vi "mainSystem.vi"() -> ()   [LabVIEW 2012, in "GUILib.lvlib"]
doc: "example for a main (top) system"
uses:
  GUILib.lvlib
  GUILib.userEventsMainType.ctl
  UtilityLib/UtilityLib.valueStatus.ctl
  UtilityLib/UtilityLib.lvlib
panel:
  in  "stop":bool
  in  "userEventsMain":T1
  in  "subSystem3":bool
  in  "userEvent":refnum<user-event>
  in  "subSystem2":bool
  in  "subSystem1":bool
  out "subSystem1state":bool
  out "subSystem3state":bool
  out "subSystem2state":bool
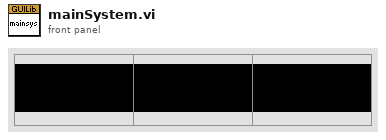
[diagram p1: front panel]
types:
  T1 = typedef "GUILib.lvlib/GUILib.userEventsMainType.ctl" = cluster{"data":string, "dataType":i32}
  T2 = typedef "UtilityLib.lvlib/UtilityLib.valueStatus.ctl" = enum16{"no info available", "stand by/off", "on", "warning", "alarm/malfunction", "not implemented", "user action required", "important information", "system default", "control default", "indicator default", "button default"}
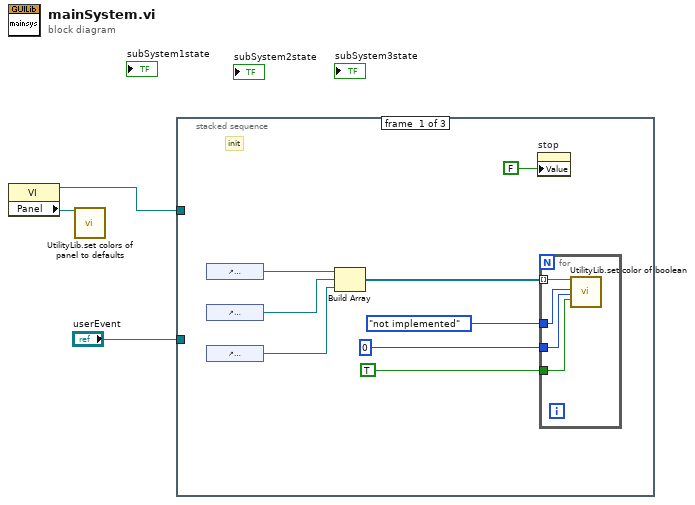
[diagram p0: block diagram]
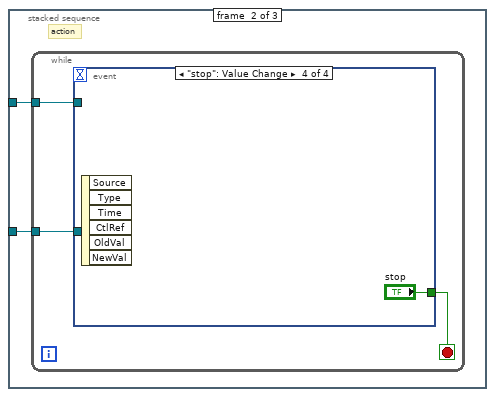
[diagram p2: hidden frame]
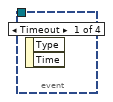
[diagram p3: hidden frame]
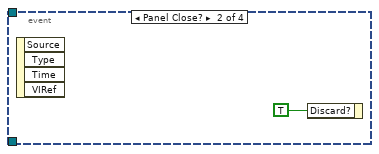
[diagram p4: hidden frame]
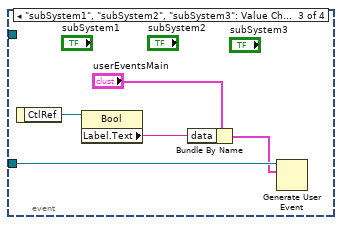
[diagram p5: hidden frame]
diagram:
  n1 = property on="Property Node" class="VI"() -> (reference out=w1:refnum<vi>, "Panel"=w2:refnum<vi>)  [unwired: 2 in, 1 out]
  n2 = call "UtilityLib.set colors of panel to defaults.vi"("Front Panel"=w2) -> ()  [unwired: 18 in, 1 out]
  n3 = stacked-sequence {
    tunnel: "userEvent" -> [_ w17 _]
    tunnel: w1 -> [_ w16 _]
    frame #0 {
      # "init"
      n4 = control-ref of="subSystem1state"() -> (w7:refnum<vi>)
      n5 = control-ref of="subSystem2state"() -> (w6:refnum<vi>)
      n6 = control-ref of="subSystem3state"() -> (w5:refnum<vi>)
      n7 = Build Array(w7, w6, w5) -> (w4:refnum<vi>[])
      n8 = property on="stop" class="Bool (strict)"("Value"=FALSE ("stop")) -> ()  [unwired: 2 in, 2 out]
      n9 = for {
        tunnel: UtilityLib.valueStatus."not implemented" ("valueStatus") -> [w15]
        tunnel: 0 ("nOfPair (0)") -> [w14]
        tunnel: TRUE ("setTRUEColor (FALSE)") -> [w13]
        tunnel: w4 -> [w12] mode=indexing
        n10 = call "UtilityLib.set color of boolean.vi"("button"=w12, "valueStatus"=w15, "nOfPair (0)"=w14, "setTRUEColor (FALSE)"=w13) -> ()  [unwired: 15 in, 1 out]
      }
    }
    frame #1 {
      # "action"
      n11 = while {
        tunnel: w17 -> [w20]
        tunnel: w16 -> [w19]
        stop <- w18 stop-if-true
        n12 = event shown="[3] \"stop\": Value Change" {
          selector: _ -> [_ _ _ _]
          dyn-events: _ -> [_ _ _ _]
          timeout: _ -> [_ _ _ _]
          tunnel: w20 -> [_ _ w26 _]
          tunnel: w19 -> [_ _ _ _]
          tunnel: [_ _ _ "stop"] -> w18
          event Timeout {
            n13 = event-data() -> ()  [unwired: 1 in, 2 out]
          }
          event Panel Close? {
            n14 = event-data() -> ()  [unwired: 1 in, 4 out]
            n15 = event-data ("Event Filter Node")("Discard?"=TRUE) -> ()  [unwired: 1 in, 1 out]
          }
          event "subSystem1", "subSystem2", "subSystem3": Value Change {
            n16 = event-data() -> ("CtlRef"=w24:refnum<vi>)  [unwired: 1 in]
            n17 = property on="Property Node" class="Bool"(reference=w24) -> ("Label.Text"=w23:string)  [unwired: 1 in, 2 out]
            n18 = Bundle By Name(cluster="userEventsMain", "data"=w23) -> (w22:T1)
            n19 = Generate User Event(user event=w26, event data cluster=w22) -> ()  [unwired: 1 in, 2 out]
          }
          event "stop": Value Change {
            n20 = event-data() -> ()  [unwired: 1 in, 6 out]
          }
        }
      }
    }
    frame #2 {
      # "deinit"
    }
  }
